vi "SUB_CHK_PQAW_ERR.vi"   [LabVIEW 2011]
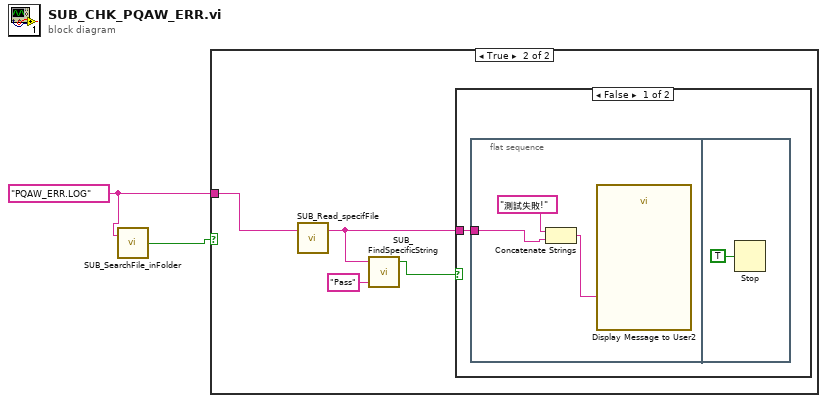
[diagram p0: block diagram]
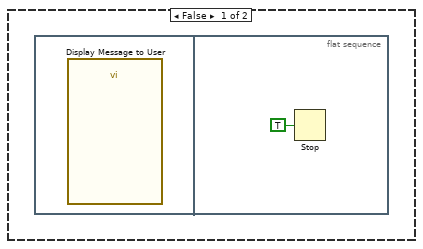
[diagram p2: hidden frame]
diagram:
  w1 = "PQAW_ERR.LOG" ("Filename to be  Deleted")
  n1 = call "SUB_SearchFile_inFolder.vi"("Search Filename in Folder"=w1) -> ("File Existing True/Flase"=w2:bool)  [unwired: 1 in]
  n2 = case shown="True" w2 {
    tunnel: w1 -> [_ w7]
    frame False {
      n3 = flat-sequence {
        frame #0 {
          n4 = call "Display Message to User"() -> ()  [unwired: 10 in, 2 out]
        }
        frame #1 {
          n5 = Stop(stop? (T)=TRUE) -> ()
        }
      }
    }
    frame True {
      n6 = call "SUB_Read_specifFile.vi"("name or relative path"=w7) -> ("text"=w4:string)  [unwired: 1 in, 1 out]
      n7 = call "SUB_FindSpecificString.vi"("Find this String"="Pass", "String data"=w4) -> ("Found"=w5:bool)  [unwired: 2 in, 1 out]
      n8 = case shown="False" w5 {
        tunnel: w4 -> [w8 _]
        frame False {
          n9 = flat-sequence {
            tunnel: w8 -> [w10]
            frame #0 {
              n10 = Concatenate Strings("測試失敗!" ("string"), w10) -> (w9:string)
              n11 = call "Display Message to User2"("Message"=w9) -> ()  [unwired: 9 in, 2 out]
            }
            frame #1 {
              n12 = Stop(stop? (T)=TRUE) -> ()
            }
          }
        }
        frame True {
        }
      }
    }
  }
